vi "_Convert Mass to DAC.vi"(5 "Calibration Table":dbl[][](array[numeric]) format="%.2f", 7 "Mass":dbl format="%.2f") -> (0 "LowerIndex":i32, 1 "UpperIndex":i32, 2 "Slope":dbl, 3 "DAC Value":dbl)   [LabVIEW 2015]
panel:
  # "Calibration table must be sorted in the mass column (1st column).\nThere should not be more than one 0 amu entry."
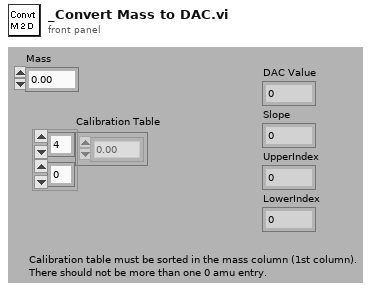
[diagram p1: front panel]
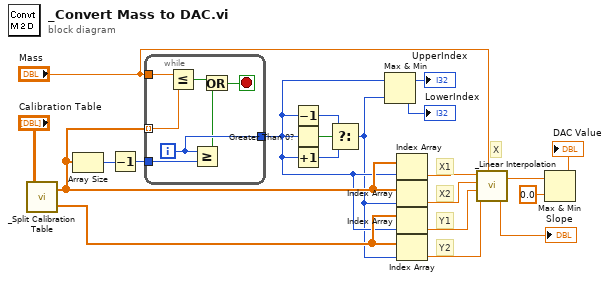
[diagram p0: block diagram]
diagram:
  # "Y2"
  # "Y1"
  # "X2"
  # "X1"
  # "X"
  n1 = call "_Split Calibration Table.vi"("Calibration"="Calibration Table") -> ("Mass"=w19:dbl[], "DAC"=w20:dbl[])
  n2 = Array Size(array=w19) -> (size(s)=w18:i32)
  n3 = Decrement(x=w18) -> (x-1=w17:i32)
  n4 = while {
    tunnel: w19 -> [w28] mode=indexing
    tunnel: "Mass" -> [w27]
    tunnel: w17 -> [w26]
    tunnel: [w25] -> w5
    i -> [w25]
    stop <- w24 stop-if-true
    n5 = Less Or Equal?(x=w27, y=w28) -> (x <= y?=w23:bool)
    n6 = Greater Or Equal?(x=w25, y=w26) -> (x >= y?=w22:bool)
    n7 = Or(x=w23, y=w22) -> (x .or. y?=w24:bool)
  }
  n8 = Decrement(x=w5) -> (x-1=w15:i32)
  n9 = Greater Than 0?(x=w5) -> (x > 0?=w16:bool)
  n10 = Increment(x=w5) -> (x+1=w14:i32)
  n11 = Select(t=w15, s=w16, f=w14) -> (s? t:f=w4:i32)
  n12 = Max & Min(x=w5, y=w4) -> (max(x,y)=→"UpperIndex":i32, min(x,y)=→"LowerIndex":i32)
  n13 = Index Array(array=w19, index=w5) -> (element=w12:dbl)
  n14 = Index Array(array=w19, index=w4) -> (element=w10:dbl)
  n15 = Index Array(array=w20, index=w5) -> (element=w9:dbl)
  n16 = Index Array(array=w20, index=w4) -> (element=w11:dbl)
  n17 = call "_Linear Interpolation.vi"("X1"=w12, "X2"=w10, "Y1"=w9, "Y2"=w11, "X"="Mass") -> ("Y"=w8:dbl, "Slope"=→"Slope":dbl)
  n18 = Max & Min(x=w8, y=0.0) -> (max(x,y)=→"DAC Value":dbl)  [unwired: 1 out]
